vi "Encrypt_Password.vi"(9 "Password in":string, 11 "Decrypt?":bool) -> (1 "Password out":string)   [LabVIEW 2013]
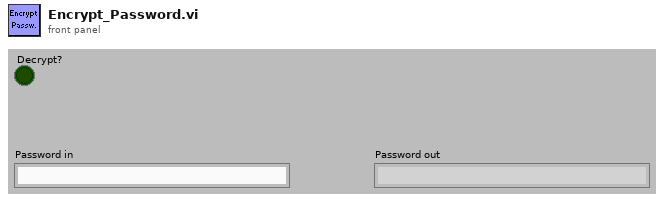
[diagram p1: front panel]
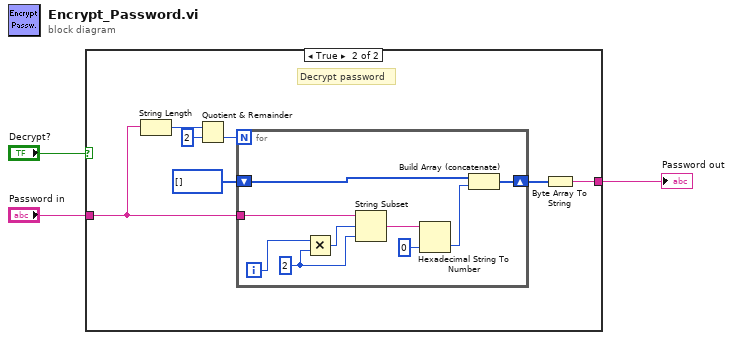
[diagram p0: block diagram]
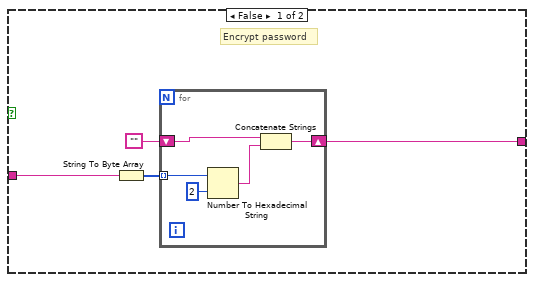
[diagram p2: hidden frame]
diagram:
  n1 = case shown="True" "Decrypt?" {
    tunnel: "Password in" -> [w7 w16]
    tunnel: [w4 w19] -> w1
    frame False {
      # "Encrypt password"
      n2 = String To Byte Array(string=w7) -> (unsigned byte array=w6:u8[])
      n3 = for {
        tunnel: w6 -> [w12] mode=indexing
        shift-right: [w9] -> w4
        shift-left: "" -> [w8]
        n4 = Number To Hexadecimal String(1:i16 2 ("width (-)"), 2:w12) -> (0:w10:string)
        n5 = Concatenate Strings(w8, w10) -> (w9:string)
      }
    }
    frame True {
      # "Decrypt password"
      n6 = String Length(string=w16) -> (length=w15:i32)
      n7 = Quotient & Remainder(x=w15, y=2) -> (floor(x/y)=w13:i32)  [unwired: 1 out]
      n8 = for {
        N: w13 -> [_]
        shift-right: [w22] -> w18
        shift-left: u8[] [] ("unsigned byte array") -> [w21]
        tunnel: w16 -> [w25]
        i -> [w27]
        w28 = 2 ("length (rest)")
        n9 = Multiply(x=w27, y=w28) -> (x*y=w26:i32)
        n10 = String Subset(string=w25, offset (0)=w26, length (rest)=w28) -> (substring=w24:string)
        n11 = Hexadecimal String To Number(string=w24, default (0uL)=u8 0 ("default (0 U32)")) -> (number=w20:u8)  [unwired: 2 out]
        n12 = Build Array (concatenate)(w21, w20) -> (w22:u8[])
      }
      n13 = Byte Array To String(unsigned byte array=w18) -> (string=w19:string)
    }
  }
  "Password out" <- w1
